vi "Dmi To Dkm.vi"(8 "error in (no error)":errorcluster, 11 "dMiles":dbl) -> (0 "error out":errorcluster, 3 "dkm":dbl)   [LabVIEW 2023, in "POSCONV.lvlib"]
doc: "Converts double miles to double kilometres (One mile is 1.609344km)...\n\ndouble DmiToDkm(double dMiles);"
uses:
  POSCONV.lvlib
  C:/Users/J Gordon/Documents/Rail Tech/TV-HR/02 - Code/Modules/POSCONV/POSCONV.dll
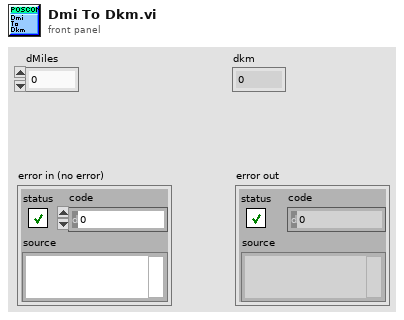
[diagram p1: front panel]
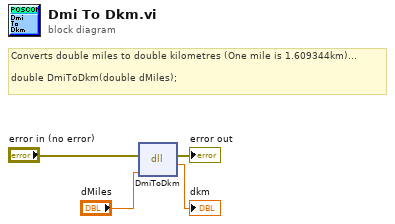
[diagram p0: block diagram]
diagram:
  # "Converts double miles to double kilometres (One mile is 1.609344km)...\n\ndouble DmiToDkm(double dMiles);"
  n1 = dll-call lib="C:/Users/J Gordon/Documents/Rail Tech/TV-HR/02 - Code/Modules/POSCONV/POSCONV.*" fn="DmiToDkm"(error in="error in (no error)", "dMiles"="dMiles") -> (error out=→"error out":errorcluster, →"dkm":dbl)  [unwired: 3 in, 1 out]
